vi "Esercitazione 3 - Termometro+.vi"() -> ()   [LabVIEW 2018]
panel:
  in  "Enum":enum16{"Celsius", "Fahrenheit", "Kelvin"}(ring)
  out "OUTPUT °F":sgl(slide) scale=-25.0..350.0
  in  "INPUT °C":sgl(slide) scale=-40.0..60.0
  # "sequenziali\nselettivi\niterativi"
  # "celsius"
  # "farenheit"
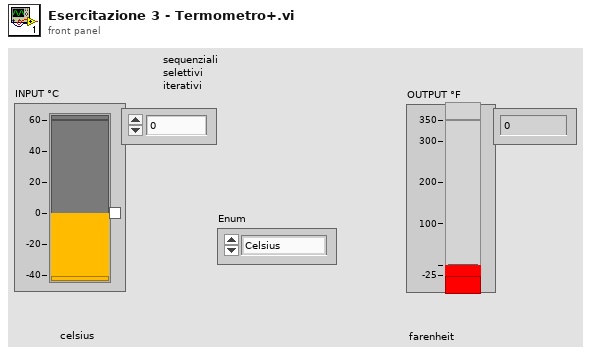
[diagram p1: front panel]
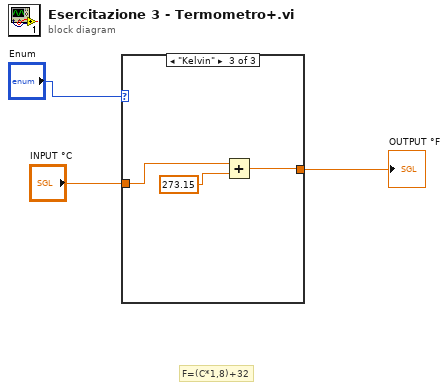
[diagram p0: block diagram]
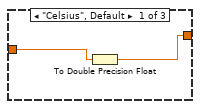
[diagram p2: hidden frame]
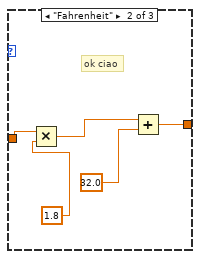
[diagram p3: hidden frame]
diagram:
  # "F=(C*1,8)+32"
  n1 = case shown="\"Kelvin\"" "Enum" {
    tunnel: "INPUT °C" -> [w4 w10 w11]
    tunnel: [w5 w7 w13] -> w2
    frame "Celsius", Default {
      n2 = To Double Precision Float(number=w4) -> (double precision float=w5:dbl)
    }
    frame "Fahrenheit" {
      # "ok ciao"
      n3 = Multiply(x=w10, y=1.8) -> (x*y=w9:dbl)
      n4 = Add(x=w9, y=32.0) -> (x+y=w7:dbl)
    }
    frame "Kelvin" {
      n5 = Add(x=w11, y=273.15) -> (x+y=w13:dbl)
    }
  }
  "OUTPUT °F" <- w2
